vi "2d_Array_sortSimplified.vi"(1 "Column to Sort on":i32=1, 2 "2D Input Array":string[][](array[string])=[["a", "5"], ["c", "31"], ["b", "2"], ["d", "4"]], 3 "Sort numerically":bool=TRUE) -> (0 "2D Ouput Array":string[][](array[string]))   [LabVIEW 2016]
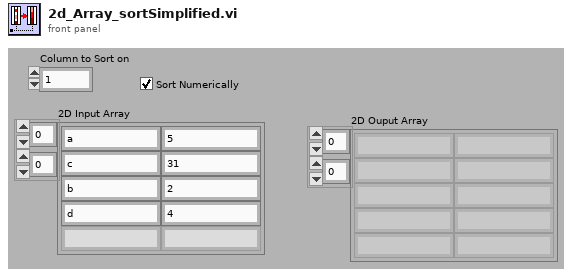
[diagram p1: front panel]
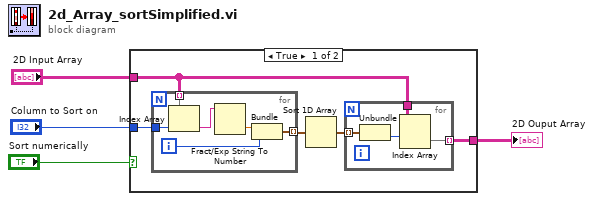
[diagram p0: block diagram]
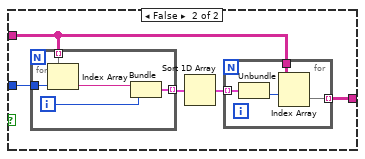
[diagram p2: hidden frame]
diagram:
  n1 = case shown="True" "Sort numerically" {
    tunnel: "Column to Sort on" -> [w7 w22]
    tunnel: "2D Input Array" -> [w6 w21]
    tunnel: [w5 w20] -> w2
    frame True {
      n2 = for {
        tunnel: w6 -> [w19] mode=indexing
        tunnel: [w16] -> w9 mode=indexing
        tunnel: w7 -> [w18]
        i -> [w17]
        n3 = Index Array(array=w19, index=w18) -> (element=w15:string)
        n4 = Fract/Exp String To Number(string=w15) -> (number=w14:dbl)  [unwired: 3 in, 1 out]
        n5 = Bundle(w14, w17) -> (w16:cluster{dbl, i32})  [unwired: 1 in]
      }
      n6 = Sort 1D Array(array=w9) -> (sorted array=w8:cluster{dbl, i32}[])
      n7 = for {
        tunnel: w8 -> [w13] mode=indexing
        tunnel: [w11] -> w5 mode=indexing
        tunnel: w6 -> [w12]
        n8 = Unbundle(w13) -> (w10:i32)  [unwired: 1 out]
        n9 = Index Array(array=w12, index (row)=w10) -> (element=w11:string[])  [unwired: 1 in]
      }
    }
    frame False {
      n10 = for {
        tunnel: w21 -> [w33] mode=indexing
        tunnel: [w30] -> w24 mode=indexing
        tunnel: w22 -> [w32]
        i -> [w31]
        n11 = Index Array(array=w33, index=w32) -> (element=w29:string)
        n12 = Bundle(w29, w31) -> (w30:cluster{string, i32})  [unwired: 1 in]
      }
      n13 = Sort 1D Array(array=w24) -> (sorted array=w23:cluster{string, i32}[])
      n14 = for {
        tunnel: w23 -> [w28] mode=indexing
        tunnel: [w26] -> w20 mode=indexing
        tunnel: w21 -> [w27]
        n15 = Unbundle(w28) -> (w25:i32)  [unwired: 1 out]
        n16 = Index Array(array=w27, index (row)=w25) -> (element=w26:string[])  [unwired: 1 in]
      }
    }
  }
  "2D Ouput Array" <- w2
